vi "readResults.vi"(8 "error in (no error)":errorcluster, 10 "address":string) -> (0 "error out":errorcluster, 3 "Results":dbl[][](array[numeric]))   [LabVIEW 2016]
uses:
  RemoteControl/Typedefs/PrivateEvents--RemoteControl.setResults.ctl
  RemoteControl/Typedefs/Remote-SMO-Commands-Enum.ctl
  RemoteControl/RemoteControl.lvclass
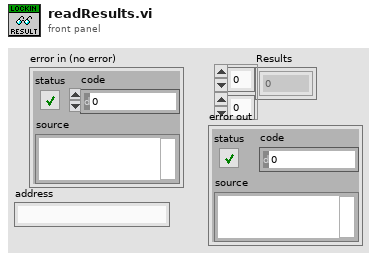
[diagram p1: front panel]
types:
  T1 = typedef "RemoteControl.lvclass/Remote-SMO-Commands-Enum.ctl" = enum16{"configAO", "configREF", "configIVmode", "configRemote", "assertTrigger", "getAO", "getAI", "getResults", "ACK", "UNK", "CLOSE"}
  T2 = typedef "RemoteControl.lvclass/PrivateEvents--RemoteControl.setResults.ctl" = dbl[][]
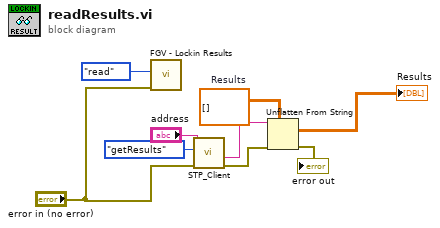
[diagram p0: block diagram]
diagram:
  w3 = T2 []  # Results
  n1 = call "FGV - Lockin Results.vi"("error in"="error in (no error)", "Function"=enum16{"write", "read"}."read") -> ()  [unwired: 4 in, 2 out]
  n2 = call "STP_Client.vi"("error in (no error)"="error in (no error)", "Command"=Remote-SMO-Commands-Enum."getResults", "address"="address") -> ("error out"=w7:errorcluster, "data received from server"=w6:string)  [unwired: 7 in]
  n3 = Unflatten From String(type=w3, binary string=w6, error in (no error)=w7) -> (value=→"Results":T2, error out=→"error out":errorcluster)  [unwired: 2 in, 1 out]
